vi "HiTech-Color-Senser_Open.vi"(7 "Timeout ms (1000)":i32=1000, 8 "Error In":errorcluster, 11 "I2C角位":tag="A/I2C") -> (0 "Error Out":errorcluster, 3 "HiTechnicColorSensorV2 Ref Out":cluster{"I2C Ref Out":T1})   [LabVIEW 2019]
uses:
  <vilib>/myRIO/Instrument Drivers/Onboard IO/I2C/I2C.lvlib
  <vilib>/myRIO/Instrument Drivers/Onboard IO/I2C/typedefs/I2C Transfer Rate.ctl
  <vilib>/myRIO/Instrument Drivers/Onboard IO/I2C/typedefs/I2C User Configuration.ctl
  <vilib>/myRIO/Instrument Drivers/Onboard IO/I2C/typedefs/I2C Configuration.ctl
  <vilib>/myRIO/Common/Instrument Driver Framework/myRIO v1.0/I2C/typedefs/I2C Channels Enum.ctl
  <vilib>/myRIO/Common/Instrument Driver Framework/Utilities/typedefs/Generic FPGA Reference.ctl
  <vilib>/myRIO/Common/Instrument Driver Framework/Utilities/typedefs/myRIO v1.0 Reference.ctl
  <vilib>/myRIO/Common/Instrument Driver Framework/Utilities/typedefs/Hardware Version Enum.ctl
  <vilib>/myRIO/Common/Instrument Driver Framework/Utilities/typedefs/myRIO Generic Hardware Reference.ctl
  <vilib>/myRIO/Instrument Drivers/Onboard IO/I2C/typedefs/I2C Reference.ctl
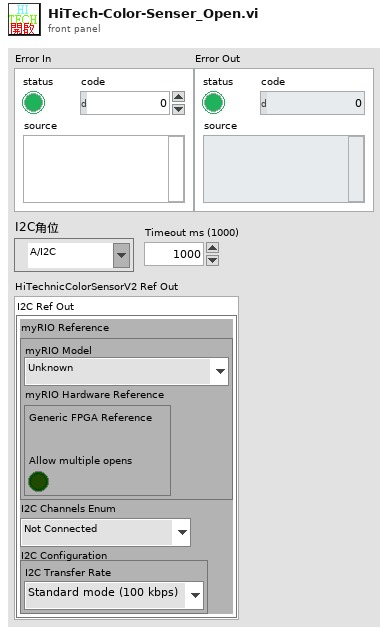
[diagram p1: front panel]
types:
  T1 = typedef "I2C.lvlib/I2C Reference.ctl" = cluster{"myRIO Reference":T2, "I2C Channels Enum":T6, "I2C Configuration":T7}
  T2 = typedef "myRIO Generic Hardware Reference.ctl" = cluster{"myRIO Model":T3, "myRIO Hardware Reference":T4}
  T3 = typedef "Hardware Version Enum.ctl" = enum16{"Unknown", "myRIO-1900", "myRIO-1950", "roboRIO", "NI ELVIS RIO CM", "ELVIS III"}
  T4 = typedef "myRIO v1.0 Reference.ctl" = cluster{"Generic FPGA Reference":T5, "Allow multiple opens":bool}
  T5 = typedef "Generic FPGA Reference.ctl" = refnum<k20>
  T6 = typedef "I2C Channels Enum.ctl" = enum16{"Not Connected", "A/I2C", "B/I2C", "I2C/I2C"}
  T7 = typedef "I2C.lvlib/I2C Configuration.ctl" = cluster{"I2C Transfer Rate":T8}
  T8 = typedef "I2C.lvlib/I2C Transfer Rate.ctl" = enum16{"Standard mode (100 kbps)", "Fast mode (400 kbps)"}
  T9 = typedef "I2C.lvlib/I2C User Configuration.ctl" = cluster{"I2C Transfer Rate":T8}
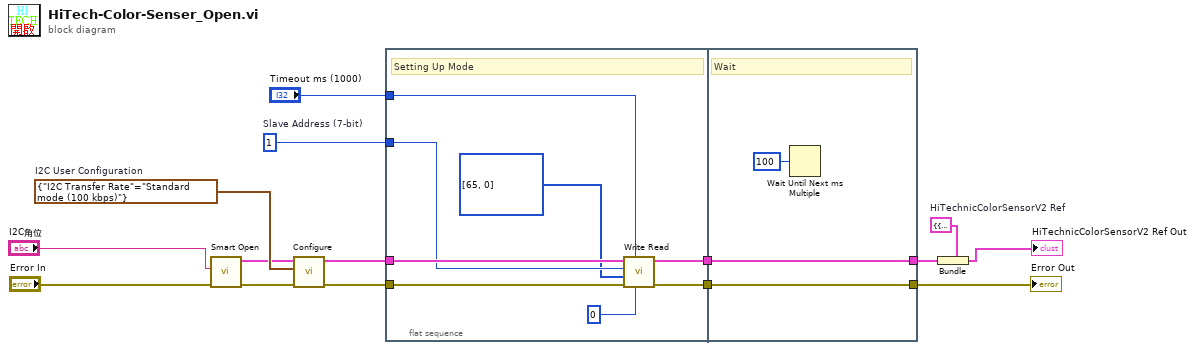
[diagram p0: block diagram]
diagram:
  w4 = u8 1  # Slave Address (7-bit)
  w5 = cluster{"I2C Ref Out":T1} {"I2C Ref Out"={"myRIO Reference"={"myRIO Model"=enum."Unknown", "myRIO Hardware Reference"={"Generic FPGA Reference"=refnum, "Allow multiple opens"=FALSE}}, "I2C Channels Enum"=enum."Not Connected", "I2C Configuration"={"I2C Transfer Rate"=enum."Standard mode (100 kbps)"}}}  # HiTechnicColorSensorV2 Ref
  w15 = T9 {"I2C Transfer Rate"=enum."Standard mode (100 kbps)"}  # I2C User Configuration
  n1 = call <vilib>:"Smart Open.vi"("error in (no error)"="Error In", "Channel Name"="I2C角位") -> ("error out"=w13:errorcluster, "I2C Ref Out"=w14:T1)  [unwired: 8 in]
  n2 = call <vilib>:"Configure.vi"("error in (no error)"=w13, "I2C User Configuration"=w15, "I2C Ref In"=w14) -> ("error out"=w11:errorcluster, "I2C Ref Out"=w12:T1)  [unwired: 7 in]
  n3 = flat-sequence {
    tunnel: w12 -> [w23]
    tunnel: w11 -> [w20]
    tunnel: [w19] -> w8
    tunnel: [w18] -> w7
    tunnel: w4 -> [w22]
    tunnel: "Timeout ms (1000)" -> [w17]
    tunnel: [w26] -> w10
    tunnel: w8 -> [w26]
    tunnel: [w24] -> w6
    tunnel: w7 -> [w24]
    frame #0 {
      # "Setting Up Mode"
      n4 = call <vilib>:"Write Read.vi"("Byte Count"=u32 0, "Timeout ms (1000)"=w17, "error in (no error)"=w20, "Bytes to Write"=u8[] [65, 0], "Slave Address (7-bit)"=w22, "I2C Ref In"=w23) -> ("error out"=w19:errorcluster, "I2C Ref Out"=w18:T1)  [unwired: 2 in, 1 out]
    }
    frame #1 {
      # "Wait"
      n5 = Wait Until Next ms Multiple(millisecond multiple=u32 100) -> ()  [unwired: 1 out]
    }
  }
  n6 = Bundle(cluster=w5, "I2C Ref Out"=w6) -> (→"HiTechnicColorSensorV2 Ref Out":cluster{"I2C Ref Out":T1})
  "Error Out" <- w10
